vi "Content-Disposition.vi"(8 "error in (no error)":errorcluster, 11 "Request in":refnum<class "Request.lvclass">) -> (0 "error out":errorcluster, 1 "Content-Type":string, 2 "Content-Disposition":T1, 3 "Request out":refnum<class "Request.lvclass">, 4 "File?":bool)   [LabVIEW 2020, in "HTTP Utils.lvlib" / "Request.lvclass"]
uses:
  Request.lvclass
  Content-Disposition.ctl
  Request.lvclass/Request.ctl
  lv-uri/URI/URI.lvlib
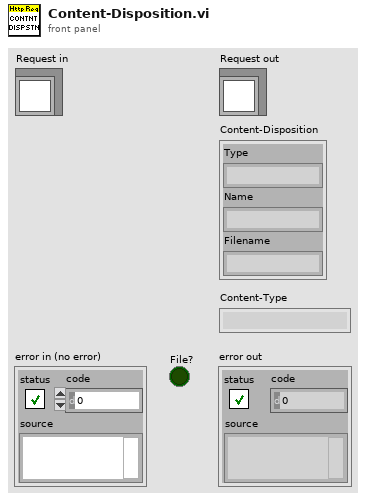
[diagram p1: front panel]
types:
  T1 = typedef "HTTP Utils.lvlib/Request.lvclass/Content-Disposition.ctl" = cluster{"Type":string, "Name":string, "Filename":string}
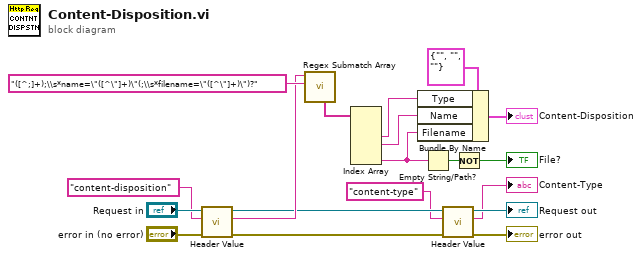
[diagram p0: block diagram]
diagram:
  n1 = call "Header Value.vi"("error in (no error)"="error in (no error)", "Header"="content-disposition", "Request in"="Request in") -> ("error out"=w4:errorcluster, "Value"=w13:string, "Request out"=w9:refnum<class "Request.lvclass">)  [unwired: 5 in, 1 out]
  n2 = call "Regex Submatch Array.vi"("regular expression"="([^;]+);\\s*name=\"([^\"]+)\"(;\\s*filename=\"([^\"]+)\")?", "string"=w13) -> ("matches"=w12:string[])  [unwired: 5 in, 4 out]
  n3 = Index Array(array=w12) -> (element #2=w11:string, element #3=w10:string, element #5=w3:string)  [unwired: 5 in, 2 out]
  n4 = Bundle By Name(cluster=T1 {"Type"="", "Name"="", "Filename"=""} ("Content-Disposition"), "Type"=w11, "Name"=w10, "Filename"=w3) -> (→"Content-Disposition":T1)
  n5 = Empty String/Path?(string/path=w3) -> (empty?=w2:bool)
  n6 = call "Header Value.vi"("error in (no error)"=w4, "Header"="content-type", "Request in"=w9) -> ("error out"=→"error out":errorcluster, "Value"=→"Content-Type":string, "Request out"=→"Request out":refnum<class "Request.lvclass">)  [unwired: 5 in, 1 out]
  n7 = Not(x=w2) -> (.not. x?=→"File?":bool)
